vi "Read Enabled Controllers.vi"(8 "error in (no error)":errorcluster, 11 "Single Channel in":refnum<class "No-Op Output.lvclass">) -> (0 "error out":errorcluster, 2 "Enabled Controllers":string[](array[string]), 3 "Single Channel out":refnum<class "No-Op Output.lvclass">)   [LabVIEW 2024, in "No-Op Output.lvclass"]
doc: "Single Channel.lvclass:Read Enabled Channels.vi\n\nThis VI returns the list of channel names that are enabled for the Single Channel class..\n\nInstrument Communication Module Version 1.0\nOctober, 2020 Original Code Consulting Davita Bird\n www.originalcode.com"
uses:
  No-Op Output.lvclass
  No-Op Output.lvclass/No-Op Output.ctl
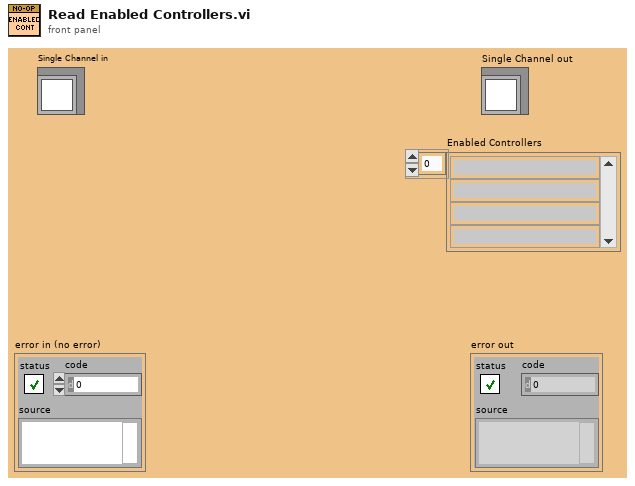
[diagram p1: front panel]
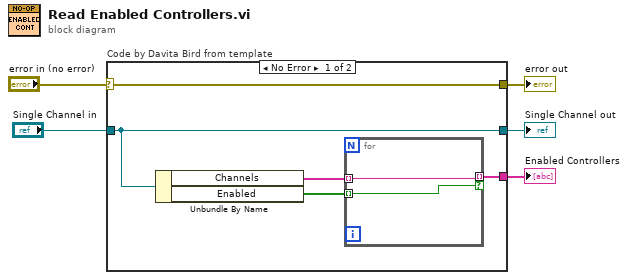
[diagram p0: block diagram]
diagram:
  n1 = case "Code by Davita Bird from template" shown="No Error" "error in (no error)" {
    selector: "error in (no error)" -> [w10 w13]
    tunnel: [w10 w13] -> w4
    tunnel: [w9 w14] -> w1
    tunnel: "Single Channel in" -> [w9 w14]
    tunnel: [w7 _] -> w3
    frame No Error {
      n2 = Unbundle By Name(w9) -> ("Channels"=w8:string[], "Enabled"=w6:bool[])
      n3 = for {
        tunnel: [w11] -> w7 mode=indexing if=w12
        tunnel: w8 -> [w11] mode=indexing
        tunnel: w6 -> [w12] mode=indexing
      }
    }
    frame Error {
    }
  }
  "error out" <- w4
  "Enabled Controllers" <- w3
  "Single Channel out" <- w1
